vi "Config IQ Modulation.vi"(0 "VISA Resource Name":refnum<visa-resource-name>, 1 "Burst Envelope (F:OFF)":bool, 2 "Burst Source (0:EXTERNAL1 DC)":enum16{"EXTERNAL1 DC", "INTERNAL BURST"}(ring), 3 "Ext I/Q Phase Polarity (T:NORM)":bool=TRUE, 5 "Status (T:ON)":bool=TRUE, 7 "I/Q Source (0:EXTERNAL I/Q)":T1(ring), 9 "High Crest Mode (F:OFF)":bool, 11 "error in (no error)":errorcluster {"code" format="%.0x"}) -> (4 "VISA Resource Name Out":refnum<visa-resource-name>, 15 "error out":errorcluster {"code" format="%.0x"})   [LabVIEW 2012, in "Agilent ESG Series.lvlib"]
doc: "This VI is used to set the I/Q modulation controls and the I/Q parameters associated with I/Q modulated signals.\n\nNotes:\n(1) This VI is for ESG-D and ESG-DP series only."
uses:
  <instrlib>/Agilent ESG Series/Agilent ESG Series.lvlib
panel:
  # "NORMAL"
  # "INVERT"
  # "ON"
  # "OFF"
  # "ON"
  # "OFF"
  # "ON"
  # "OFF"
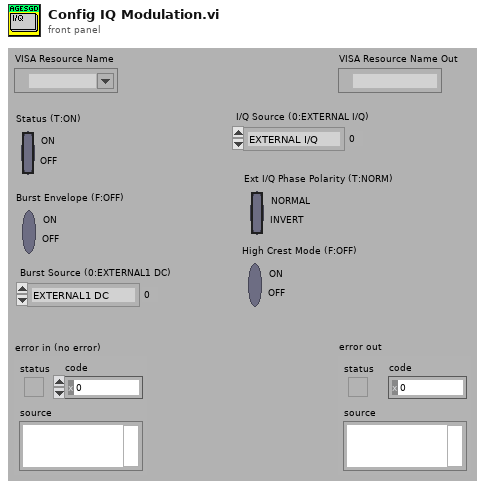
[diagram p1: front panel]
types:
  T1 = enum16{"EXTERNAL I/Q", "INTERNAL I/Q", "BBG1", "EXT600", "OFF"}
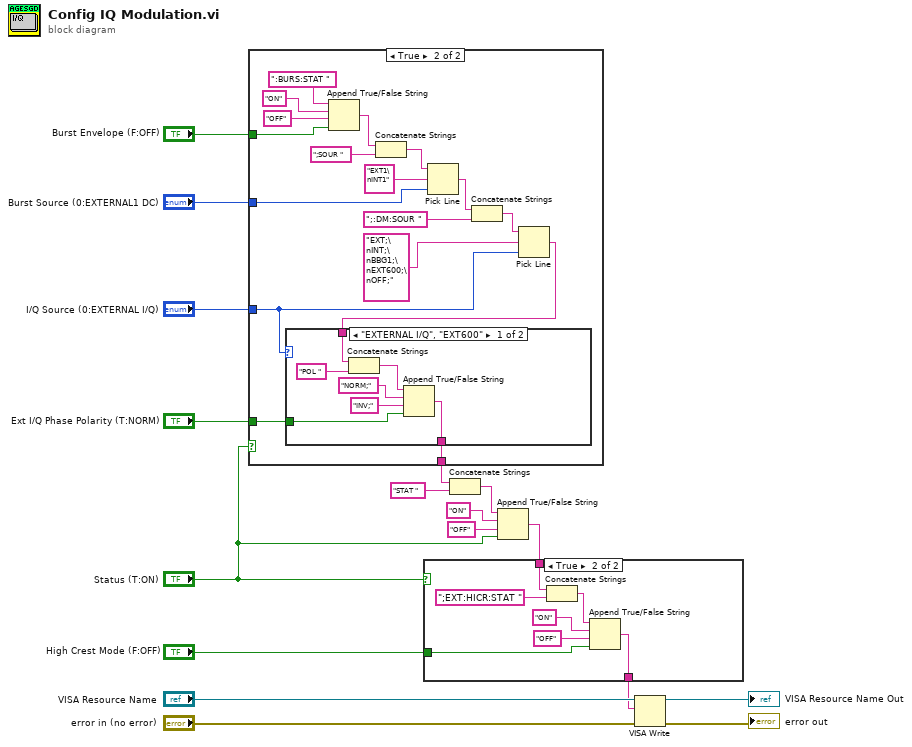
[diagram p0: block diagram]
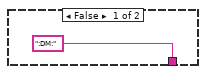
[diagram p2: hidden frame]
diagram:
  n1 = case shown="True" "Status (T:ON)" {
    tunnel: [":DM:" ("string (\"\")") w25] -> w4
    tunnel: "Ext I/Q Phase Polarity (T:NORM)" -> [_ w24]
    tunnel: "I/Q Source (0:EXTERNAL I/Q)" -> [_ w19]
    tunnel: "Burst Source (0:EXTERNAL1 DC)" -> [_ w23]
    tunnel: "Burst Envelope (F:OFF)" -> [_ w22]
    frame False {
    }
    frame True {
      n2 = Append True/False String(1:w22, 2:"OFF" ("false string"), 3:"ON" ("true string"), 4:":BURS:STAT ") -> (0:w29:string)
      n3 = Concatenate Strings(w29, ";SOUR ") -> (w30:string)
      n4 = Pick Line(string ("")=w30, multi-line string="EXT1\nINT1", line index=w23) -> (output string=w32:string)
      n5 = Concatenate Strings(w32, ";:DM:SOUR " ("string (\"\")")) -> (w34:string)
      n6 = Pick Line(string ("")=w34, multi-line string="EXT;\nINT;\nBBG1;\nEXT600;\nOFF;", line index=w19) -> (output string=w35:string)
      n7 = case shown="\"EXTERNAL I/Q\", \"EXT600\"" w19 {
        tunnel: w35 -> [w39 w43]
        tunnel: [w37 w43] -> w25
        tunnel: w24 -> [w36 _]
        frame "EXTERNAL I/Q", "EXT600" {
          n8 = Concatenate Strings(w39, "POL " ("string (\"\")")) -> (w38:string)
          n9 = Append True/False String(1:w36, 2:"INV;" ("false string"), 3:"NORM;" ("true string"), 4:w38) -> (0:w37:string)
        }
        frame "INTERNAL I/Q", "BBG1", "OFF" {
        }
      }
    }
  }
  n10 = Concatenate Strings(w4, "STAT ") -> (w12:string)
  n11 = Append True/False String(1:"Status (T:ON)", 2:"OFF" ("false string"), 3:"ON" ("true string"), 4:w12) -> (0:w5:string)
  n12 = case shown="True" "Status (T:ON)" {
    tunnel: w5 -> [w44 w48]
    tunnel: [w44 w46] -> w1
    tunnel: "High Crest Mode (F:OFF)" -> [_ w45]
    frame False {
    }
    frame True {
      n13 = Concatenate Strings(w48, ";EXT:HICR:STAT " ("string (\"\")")) -> (w47:string)
      n14 = Append True/False String(1:w45, 2:"OFF" ("false string"), 3:"ON" ("true string"), 4:w47) -> (0:w46:string)
    }
  }
  n15 = VISA Write(VISA resource name="VISA Resource Name", write buffer=w1, error in (no error)="error in (no error)") -> (VISA resource name out=→"VISA Resource Name Out":refnum<visa-resource-name>, error out=→"error out":errorcluster)  [unwired: 1 out]
